vi "close.vi"(8 "error in (no error)":errorcluster, 11 "interface in":refnum<class "interface.lvclass">) -> (0 "error out":errorcluster, 3 "interface out":refnum<class "interface.lvclass">)   [LabVIEW 2015, in "example_01.lvlib" / "functional.lvlib" / "interface.lvclass"]
uses:
  interface.lvclass
  interface.lvclass/interface.ctl
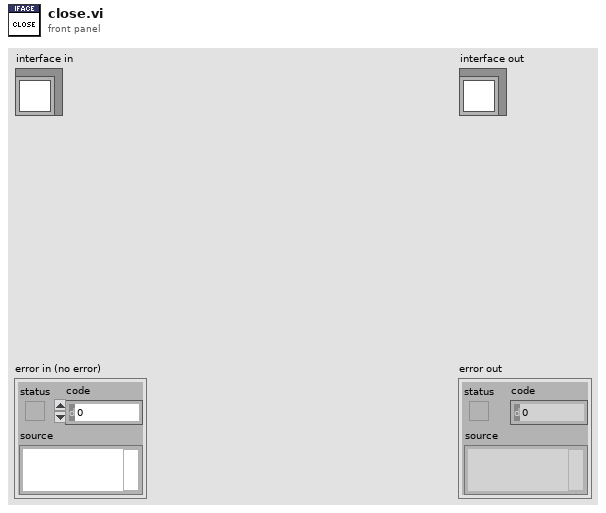
[diagram p1: front panel]
types:
  T1 = typedef "example_01.lvlib/functional.lvlib/interface.lvclass/vi_reference.ctl" = refnum<vi>
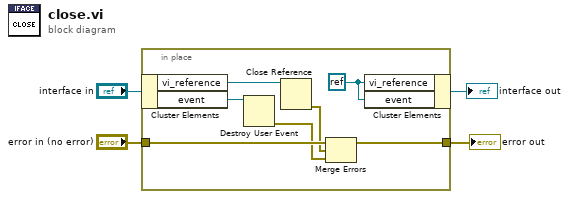
[diagram p0: block diagram]
diagram:
  n1 = in-place {
    in-place-border: "error in (no error)" -> [w11]
    in-place-border: [w7] -> w2
    w10 = refnum<k0> refnum
    n2 = in-place-cluster #1("interface in") -> ("vi_reference"=w9:T1, "event"=w8:refnum<user-event>)
    n3 = Destroy User Event(user event=w8) -> (error out=w5:errorcluster)  [unwired: 1 in]
    n4 = Close Reference(reference=w9) -> (error out=w6:errorcluster)  [unwired: 1 in]
    n5 = Merge Errors(w11, w6, w5) -> (w7:errorcluster)
    n6 = in-place-cluster #1("vi_reference"=w10, "event"=w10) -> (→"interface out":refnum<class "interface.lvclass">)
  }
  "error out" <- w2
